vi "terminate.vi"(8 "error in (no error)":errorcluster, 11 "GenericPlugin in":refnum<class "ClockMT120808DAQmxSimple.lvclass">) -> (0 "error out":errorcluster, 3 "GenericPlugin out":refnum<class "ClockMT120808DAQmxSimple.lvclass">)   [LabVIEW 2010, in "ClockMT120808DAQmxSimple.lvclass"]
doc: "The dynamic dispatch version of this VI terminates the plug-in object by releasing all of its resources."
uses:
  ClockMT120808DAQmxSimple.lvclass
  ClockMT120808DAQmxSimple.lvclass/ClockMT120808DAQmxSimple.ctl
  GenericClock/GenericClock/GenericClock.lvclass
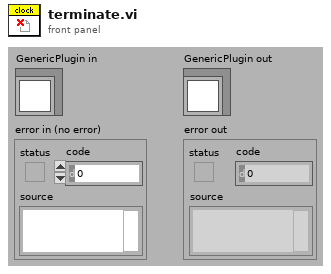
[diagram p1: front panel]
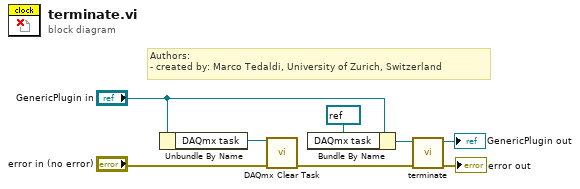
[diagram p0: block diagram]
diagram:
  # "Authors: \n- created by: Marco Tedaldi, University of Zurich, Switzerland"
  n1 = Unbundle By Name("GenericPlugin in") -> ("DAQmx task"=w5:refnum<k21>)
  n2 = call <vilib>:"DAQmx Clear Task.vi"("task in"=w5, "error in"="error in (no error)") -> ("error out"=w2:errorcluster)  [unwired: 13 in]
  n3 = Bundle By Name(cluster="GenericPlugin in", "DAQmx task"=refnum<k21> refnum) -> (w6:refnum<class "ClockMT120808DAQmxSimple.lvclass">)
  n4 = call-parent "terminate.vi"("error in (no error)"=w2, "GenericPlugin in"=w6) -> ("error out"=→"error out":errorcluster, "GenericPlugin out"=→"GenericPlugin out":refnum<class "ClockMT120808DAQmxSimple.lvclass">)  [unwired: 8 in]
